vi "test_Packet_SimplePipelineResult.vi"(8 "error in (no error)":errorcluster) -> (0 "error out":errorcluster, 3 "Test Passed":bool)   [LabVIEW 2019]
uses:
  <vilib>/Rock Robotics/WPI/ThirdParty/JAS_Junk/TrajLib/VI/Quaternion_New.vi
  <vilib>/Rock Robotics/WPI/ThirdParty/PhotonVisionLib/SubVI/Packet_encode_ByteI8.vi
  <vilib>/Rock Robotics/WPI/ThirdParty/PhotonVisionLib/SubVI/PhotonMultiTargetPNPResult_pack.vi
  <vilib>/Rock Robotics/WPI/ThirdParty/PhotonVisionLib/SubVI/PhotonPipelineResult_GetMetadata.vi
  <vilib>/Rock Robotics/WPI/ThirdParty/PhotonVisionLib/SubVI/PhotonPipelineMetadata_Pack.vi
  <vilib>/Rock Robotics/WPI/ThirdParty/PhotonVisionLib/SubVI/PhotonTrackedTarget_Pack.vi
  <vilib>/Rock Robotics/WPI/ThirdParty/PhotonVisionLib/SubVI/Packet_decode_ByteI8.vi
  <vilib>/Rock Robotics/WPI/ThirdParty/PhotonVisionLib/SubVI/PhotonTrackedTarget_Unpack.vi
  <vilib>/Rock Robotics/WPI/ThirdParty/PhotonVisionLib/SubVI/PhotonMultiTargetPNPResult_unpack.vi
  <vilib>/Rock Robotics/WPI/ThirdParty/PhotonVisionLib/SubVI/PhotonPipelineMetadata_Unpack.vi
  <vilib>/Rock Robotics/WPI/ThirdParty/PhotonVisionLib/SubVI/PhotonTrackedTarget_Equals.vi
  <vilib>/Rock Robotics/WPI/ThirdParty/PhotonVisionLib/SubVI/PhotonPipelineMetadata_Equals.vi
  <vilib>/Rock Robotics/WPI/ThirdParty/PhotonVisionLib/SubVI/PhotonMultiTargetPNPResult_Equals.vi
  <vilib>/Rock Robotics/WPI/ThirdParty/PhotonVisionLib/SubVI/Packet_encode_Boolean.vi
  <vilib>/Rock Robotics/WPI/ThirdParty/PhotonVisionLib/SubVI/PhotonPNPResult_pack.vi
  <vilib>/Rock Robotics/WPI/ThirdParty/PhotonVisionLib/SubVI/Packet_encode_Int16.vi
  <vilib>/Rock Robotics/WPI/ThirdParty/PhotonVisionLib/SubVI/Packet_encode_Int64.vi
  <vilib>/Rock Robotics/WPI/ThirdParty/PhotonVisionLib/SubVI/PhotonTrackedTarget_GetArea.vi
  <vilib>/Rock Robotics/WPI/ThirdParty/PhotonVisionLib/SubVI/PhotonTrackedTarget_GetBestCameraToTarget.vi
  <vilib>/Rock Robotics/WPI/ThirdParty/PhotonVisionLib/SubVI/PhotonTrackedTarget_GetMinAreaRectCorners.vi
  <vilib>/Rock Robotics/WPI/ThirdParty/PhotonVisionLib/SubVI/PhotonTrackedTarget_GetPitch.vi
  <vilib>/Rock Robotics/WPI/ThirdParty/PhotonVisionLib/SubVI/PhotonTrackedTarget_GetSkew.vi
  <vilib>/Rock Robotics/WPI/ThirdParty/PhotonVisionLib/SubVI/PhotonTrackedTarget_GetYaw.vi
  <vilib>/Rock Robotics/WPI/ThirdParty/PhotonVisionLib/SubVI/Packet_encode_FLT64.vi
  <vilib>/Rock Robotics/WPI/ThirdParty/PhotonVisionLib/SubVI/PhotonTrackedTarget_GetAltCameraToTarget.vi
  <vilib>/Rock Robotics/WPI/ThirdParty/PhotonVisionLib/SubVI/Packet_encode_Transform3d.vi
  <vilib>/Rock Robotics/WPI/ThirdParty/PhotonVisionLib/SubVI/PhotonTrackedTarget_GetFiducialId.vi
  <vilib>/Rock Robotics/WPI/ThirdParty/PhotonVisionLib/SubVI/Packet_encode_Int32.vi
  <vilib>/Rock Robotics/WPI/ThirdParty/PhotonVisionLib/SubVI/PhotonTrackedTarget_GetPoseAmbiguity.vi
  <vilib>/Rock Robotics/WPI/ThirdParty/PhotonVisionLib/SubVI/PhotonTrackedTarget_GetDetectedCorners.vi
  <vilib>/Rock Robotics/WPI/ThirdParty/PhotonVisionLib/SubVI/Packet_encode_FLT32.vi
  <vilib>/Rock Robotics/WPI/ThirdParty/PhotonVisionLib/SubVI/PhotonTrackedTarget_GetDetectedObjectClassID.vi
  <vilib>/Rock Robotics/WPI/ThirdParty/PhotonVisionLib/SubVI/PhotonTrackedTarget_GetDetectedObjectConfidence.vi
  <vilib>/Rock Robotics/WPI/ThirdParty/PhotonVisionLib/SubVI/Packet_encode_TargetCornerArray.vi
  <vilib>/Rock Robotics/WPI/ThirdParty/PhotonVisionLib/SubVI/Packet_decode_Flt64.vi
  <vilib>/Rock Robotics/WPI/ThirdParty/PhotonVisionLib/SubVI/Packet_decode_Int32.vi
  <vilib>/Rock Robotics/WPI/ThirdParty/PhotonVisionLib/SubVI/Packet_decode_Transform3d.vi
  <vilib>/Rock Robotics/WPI/ThirdParty/PhotonVisionLib/SubVI/Packet_decode_Flt32.vi
  <vilib>/Rock Robotics/WPI/ThirdParty/PhotonVisionLib/SubVI/Packet_decode_TargetCornerArray.vi
  <vilib>/Rock Robotics/WPI/ThirdParty/PhotonVisionLib/SubVI/Packet_decode_Boolean.vi
  <vilib>/Rock Robotics/WPI/ThirdParty/PhotonVisionLib/SubVI/PhotonPNPResult_unpack.vi
  <vilib>/Rock Robotics/WPI/ThirdParty/PhotonVisionLib/SubVI/PhotonMultiTargetPNPResult_New.vi
  <vilib>/Rock Robotics/WPI/ThirdParty/PhotonVisionLib/SubVI/Packet_decode_Int16.vi
  <vilib>/Rock Robotics/WPI/ThirdParty/PhotonVisionLib/SubVI/Packet_decode_Int64.vi
  <vilib>/Rock Robotics/WPI/ThirdParty/JAS_Junk/TrajLib/VI/Transform3d_Equals.vi
  <vilib>/Rock Robotics/WPI/ThirdParty/PhotonVisionLib/SubVI/TargetCorner_Equals.vi
  <vilib>/Rock Robotics/WPI/ThirdParty/PhotonVisionLib/SubVI/PhotonPNPResult_Equals.vi
  <vilib>/Rock Robotics/WPI/ThirdParty/JAS_Junk/TrajLib/VI/Transform3d_GetRotation3d.vi
  <vilib>/Rock Robotics/WPI/ThirdParty/JAS_Junk/TrajLib/VI/Transform3d_GetTranslation3d.vi
  <vilib>/Rock Robotics/WPI/ThirdParty/JAS_Junk/TrajLib/VI/Translation3d_ToTranslation2d.vi
  <vilib>/Rock Robotics/WPI/ThirdParty/JAS_Junk/TrajLib/VI/Rotation3d_ToRotation2d.vi
  <vilib>/Rock Robotics/WPI/ThirdParty/JAS_Junk/TrajLib/Transform2d_Create_TransRot.vi
  <vilib>/Rock Robotics/WPI/ThirdParty/JAS_Junk/TrajLib/VI/Transform3d_GetXYZ.vi
  <vilib>/Rock Robotics/WPI/ThirdParty/JAS_Junk/TrajLib/VI/Rotation3d_GetQuaterion.vi
  <vilib>/Rock Robotics/WPI/ThirdParty/JAS_Junk/TrajLib/VI/Quaternion_Get_All.vi
  <vilib>/Rock Robotics/WPI/ThirdParty/PhotonVisionLib/SubVI/TargetCorner_GetAll.vi
  <vilib>/Rock Robotics/WPI/ThirdParty/JAS_Junk/TrajLib/VI/Rotation3d_Create_Quaternion.vi
  <vilib>/Rock Robotics/WPI/ThirdParty/PhotonVisionLib/SubVI/PhotonPNPResult_New.vi
  <vilib>/Rock Robotics/WPI/ThirdParty/JAS_Junk/TrajLib/VI/Rotation3d_Equals.vi
  <vilib>/Rock Robotics/WPI/ThirdParty/JAS_Junk/TrajLib/VI/Translation3d_Equals.vi
  <vilib>/Rock Robotics/WPI/ThirdParty/JAS_Junk/TrajLib/Translation2d_Create.vi
  <vilib>/Rock Robotics/WPI/ThirdParty/JAS_Junk/TrajLib/Rotation2d_CreateAngle.vi
  <vilib>/Rock Robotics/WPI/ThirdParty/JAS_Junk/TrajLib/VI/Rotation3d_GetXYZ.vi
  <vilib>/Rock Robotics/WPI/ThirdParty/JAS_Junk/TrajLib/VI/Translation3d_GetXYZ.vi
  <vilib>/Rock Robotics/WPI/ThirdParty/JAS_Junk/TrajLib/VI/Quaternion_Normalize.vi
  <vilib>/Rock Robotics/WPI/ThirdParty/JAS_Junk/TrajLib/VI/Quaternion_Equals.vi
  <vilib>/Rock Robotics/WPI/ThirdParty/JAS_Junk/TrajLib/VI/Quaternion_New_Default.vi
  <vilib>/Rock Robotics/WPI/ThirdParty/JAS_Junk/TrajLib/VI/Quaternion_Get_Vect.vi
  <vilib>/Rock Robotics/WPI/ThirdParty/JAS_Junk/TrajLib/VI/Quaternion_Get_W.vi
  <vilib>/Rock Robotics/WPI/ThirdParty/PhotonVisionLib/PhotonVisionLib.lvlib
  <vilib>/Rock Robotics/WPI/ThirdParty/PhotonVisionLib/TypeDef/TargetCornerType.ctl
  <vilib>/Rock Robotics/WPI/ThirdParty/PhotonVisionLib/TypeDef/PhotonTrackedTargetType.ctl
  <vilib>/Rock Robotics/WPI/ThirdParty/JAS_Junk/TrajLib/TypeDef/QUATERNION.ctl
  <vilib>/Rock Robotics/WPI/ThirdParty/JAS_Junk/TrajLib/Trajectory_Library.lvlib
  <vilib>/Rock Robotics/WPI/ThirdParty/JAS_Junk/TrajLib/TypeDef/ROTATION3D.ctl
  <vilib>/Rock Robotics/WPI/ThirdParty/JAS_Junk/TrajLib/TypeDef/TRANSLATION3D.ctl
  <vilib>/Rock Robotics/WPI/ThirdParty/JAS_Junk/TrajLib/TypeDef/TRANSFORM3D.ctl
panel:
  out "Parsing Issue1":bool
  out "Parsing Issue2":bool
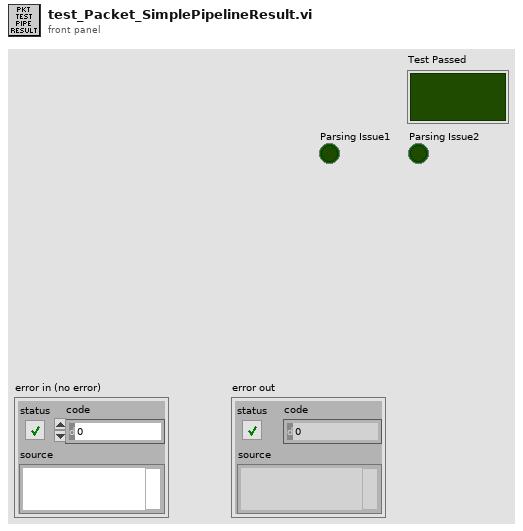
[diagram p1: front panel]
types:
  T1 = typedef "PhotonVisionLib.lvlib/PhotonTrackedTargetType.ctl" = cluster{"Yaw":dbl, "Pitch":dbl, "Area":dbl, "Skew":dbl, "MinAreaRectCorners":T2[], "BestCameraToTarget":T3, "FiducialId":i32, "AltCameraToTarget":T3, "PoseAmbiguity":dbl, "DetectedCorners":T2[], "ObjDetectId":i32, "ObjDetectConf":sgl}
  T2 = typedef "PhotonVisionLib.lvlib/TargetCornerType.ctl" = cluster{"X":dbl, "Y":dbl}
  T3 = typedef "Trajectory_Library.lvlib/TRANSFORM3D.ctl" = cluster{"TRANSLATION3D":T4, "ROTATION3D":T5, "XF":bool}
  T4 = typedef "Trajectory_Library.lvlib/TRANSLATION3D.ctl" = cluster{"X":dbl, "Y":dbl, "Z":dbl}
  T5 = typedef "Trajectory_Library.lvlib/ROTATION3D.ctl" = cluster{"Q_quaternion":T6}
  T6 = typedef "Trajectory_Library.lvlib/QUATERNION.ctl" = cluster{"R":dbl, "V":dbl[]}
  T7 = typedef "PhotonVisionLib.lvlib/PhotonPipelineMetadataType.ctl" = cluster{"CaptureTimestampMicros":i64, "PublishTimestampMicros":i64, "SequenceID":i64, "TimeSinceLastPong":i64}
  T8 = typedef "PhotonVisionLib.lvlib/PhotonPipelineResultType.ctl" = cluster{"Targets":T1[], "PhotonMultiTargetPNPResult":T9, "PhotonPipelineMetadata":T7}
  T9 = typedef "PhotonVisionLib.lvlib/PhotonMultiTargetPNPResultType.ctl" = cluster{"PhotonPNPResult":T10, "FiducialIDsUsed":i16[]}
  T10 = typedef "PhotonVisionLib.lvlib/PhotonPNPResultType.ctl" = cluster{"IsPresent":bool, "bestReprojErr":dbl, "altReprojErr":dbl, "ambiguity":dbl, "Best":T3, "Alt":T3}
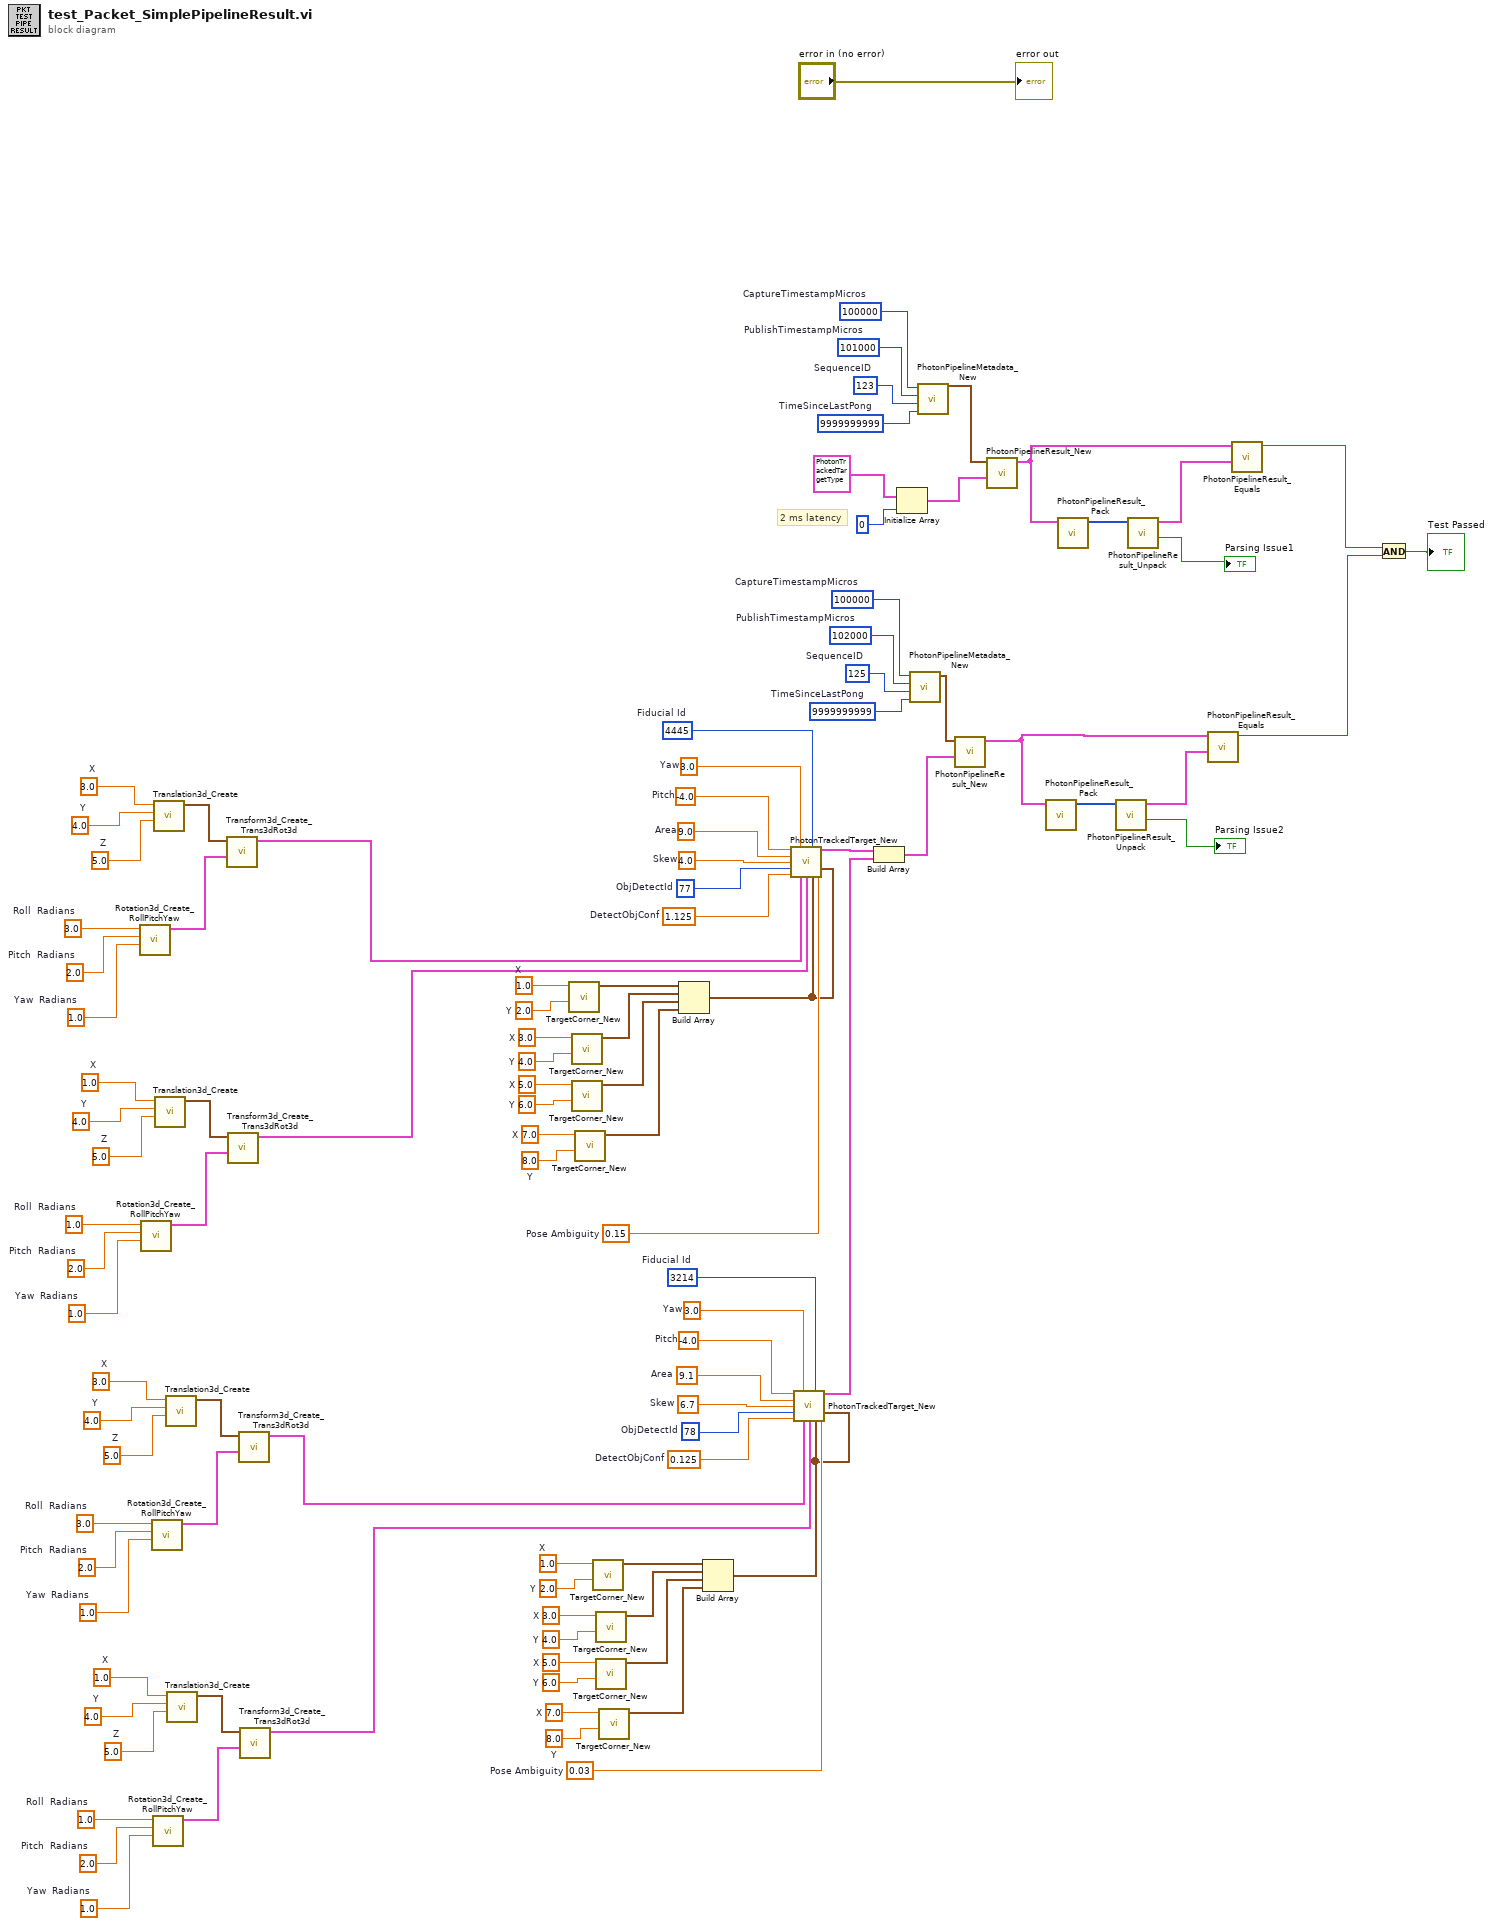
[diagram p0: block diagram]
diagram:
  w2 = sgl 0.125  # DetectObjConf
  w3 = 78  # ObjDetectId
  w4 = sgl 1.125  # DetectObjConf
  w5 = 77  # ObjDetectId
  w11 = 7.0  # X
  w12 = 8.0  # Y
  w13 = 5.0  # X
  w14 = 6.0  # Y
  w15 = 3.0  # X
  w16 = 4.0  # Y
  w17 = 1.0  # X
  w18 = 2.0  # Y
  w21 = i64 100000  # CaptureTimestampMicros
  w22 = i64 101000  # PublishTimestampMicros
  w23 = i64 123  # SequenceID
  w24 = i64 9999999999  # TimeSinceLastPong
  w26 = i64 100000  # CaptureTimestampMicros
  w27 = i64 102000  # PublishTimestampMicros
  w28 = i64 125  # SequenceID
  w29 = i64 9999999999  # TimeSinceLastPong
  w36 = 1.0  # Roll  Radians
  w35 = 2.0  # Pitch  Radians
  w34 = 1.0  # Yaw  Radians
  w38 = 1.0  # X
  w39 = 4.0  # Y
  w40 = 5.0  # Z
  w44 = 3.0  # Roll  Radians
  w43 = 2.0  # Pitch  Radians
  w42 = 1.0  # Yaw  Radians
  w46 = 3.0  # X
  w47 = 4.0  # Y
  w48 = 5.0  # Z
  w54 = 1.0  # Roll  Radians
  w53 = 2.0  # Pitch  Radians
  w52 = 1.0  # Yaw  Radians
  w56 = 1.0  # X
  w57 = 4.0  # Y
  w58 = 5.0  # Z
  w62 = 3.0  # Roll  Radians
  w61 = 2.0  # Pitch  Radians
  w60 = 1.0  # Yaw  Radians
  w64 = 3.0  # X
  w65 = 4.0  # Y
  w66 = 5.0  # Z
  w67 = 0.15  # Pose Ambiguity
  w68 = 0.03  # Pose Ambiguity
  w69 = 4445  # Fiducial Id
  w70 = 3214  # Fiducial Id
  w86 = -4.0  # Pitch
  w87 = 9.1  # Area
  w88 = 6.7  # Skew
  w89 = 3.0  # Yaw
  w90 = -4.0  # Pitch
  w91 = 9.0  # Area
  w92 = 4.0  # Skew
  w93 = 3.0  # Yaw
  w98 = 7.0  # X
  w99 = 8.0  # Y
  w100 = 5.0  # X
  w101 = 6.0  # Y
  w102 = 3.0  # X
  w103 = 4.0  # Y
  w104 = 1.0  # X
  w105 = 2.0  # Y
  # "2 ms latency"
  n1 = call <vilib>:"Rotation3d_Create_RollPitchYaw.vi"("Yaw"=w60, "Pitch"=w61, "Roll"=w62) -> ("Rotation3d"=w59:T5)  [unwired: 8 in]
  n2 = call <vilib>:"Rotation3d_Create_RollPitchYaw.vi"("Yaw"=w52, "Pitch"=w53, "Roll"=w54) -> ("Rotation3d"=w51:T5)  [unwired: 8 in]
  n3 = call <vilib>:"Rotation3d_Create_RollPitchYaw.vi"("Yaw"=w42, "Pitch"=w43, "Roll"=w44) -> ("Rotation3d"=w41:T5)  [unwired: 8 in]
  n4 = call <vilib>:"Rotation3d_Create_RollPitchYaw.vi"("Yaw"=w34, "Pitch"=w35, "Roll"=w36) -> ("Rotation3d"=w33:T5)  [unwired: 8 in]
  n5 = call <vilib>:"Translation3d_Create.vi"("Z"=w66, "Y"=w65, "X"=w64) -> ("TRANSLATION3D"=w63:T4)  [unwired: 8 in]
  n6 = call <vilib>:"Translation3d_Create.vi"("Z"=w58, "Y"=w57, "X"=w56) -> ("TRANSLATION3D"=w55:T4)  [unwired: 8 in]
  n7 = call <vilib>:"Translation3d_Create.vi"("Z"=w48, "Y"=w47, "X"=w46) -> ("TRANSLATION3D"=w45:T4)  [unwired: 8 in]
  n8 = call <vilib>:"Translation3d_Create.vi"("Z"=w40, "Y"=w39, "X"=w38) -> ("TRANSLATION3D"=w37:T4)  [unwired: 8 in]
  n9 = call <vilib>:"Transform3d_Create_Trans3dRot3d.vi"("Rotation3d"=w59, "Translation3d"=w63) -> ("Transform3d"=w50:T3)  [unwired: 9 in]
  n10 = call <vilib>:"Transform3d_Create_Trans3dRot3d.vi"("Rotation3d"=w51, "Translation3d"=w55) -> ("Transform3d"=w49:T3)  [unwired: 9 in]
  n11 = call <vilib>:"Transform3d_Create_Trans3dRot3d.vi"("Rotation3d"=w41, "Translation3d"=w45) -> ("Transform3d"=w32:T3)  [unwired: 9 in]
  n12 = call <vilib>:"Transform3d_Create_Trans3dRot3d.vi"("Rotation3d"=w33, "Translation3d"=w37) -> ("Transform3d"=w31:T3)  [unwired: 9 in]
  n13 = call <vilib>:"TargetCorner_New.vi"("Y"=w105, "X"=w104) -> ("TargetCorner"=w97:T2)  [unwired: 9 in]
  n14 = call <vilib>:"TargetCorner_New.vi"("Y"=w103, "X"=w102) -> ("TargetCorner"=w96:T2)  [unwired: 9 in]
  n15 = call <vilib>:"TargetCorner_New.vi"("Y"=w101, "X"=w100) -> ("TargetCorner"=w95:T2)  [unwired: 9 in]
  n16 = call <vilib>:"TargetCorner_New.vi"("Y"=w99, "X"=w98) -> ("TargetCorner"=w94:T2)  [unwired: 9 in]
  n17 = call <vilib>:"TargetCorner_New.vi"("Y"=w18, "X"=w17) -> ("TargetCorner"=w10:T2)  [unwired: 9 in]
  n18 = call <vilib>:"TargetCorner_New.vi"("Y"=w16, "X"=w15) -> ("TargetCorner"=w9:T2)  [unwired: 9 in]
  n19 = call <vilib>:"TargetCorner_New.vi"("Y"=w14, "X"=w13) -> ("TargetCorner"=w8:T2)  [unwired: 9 in]
  n20 = call <vilib>:"TargetCorner_New.vi"("Y"=w12, "X"=w11) -> ("TargetCorner"=w7:T2)  [unwired: 9 in]
  n21 = Build Array(w97, w96, w95, w94) -> (w30:T2[])
  n22 = Build Array(w10, w9, w8, w7) -> (w6:T2[])
  n23 = call <vilib>:"PhotonTrackedTarget_New.vi"("Pitch"=w90, "Yaw"=w93, "Fiducial Id"=w69, "Area"=w91, "Skew"=w92, "ObjDetectId"=w5, "DetectedCorners"=w30, "DetectObjConf"=w4, "BestCameraToTarget"=w50, "AltCameraToTarget"=w49, "MinAreaRectCorners"=w30, "Pose Ambiguity"=w67) -> ("TrackedTarget"=w85:T1)  [unwired: 3 in]
  n24 = call <vilib>:"PhotonTrackedTarget_New.vi"("Pitch"=w86, "Yaw"=w89, "Fiducial Id"=w70, "Area"=w87, "Skew"=w88, "ObjDetectId"=w3, "DetectedCorners"=w6, "DetectObjConf"=w2, "BestCameraToTarget"=w32, "AltCameraToTarget"=w31, "MinAreaRectCorners"=w6, "Pose Ambiguity"=w68) -> ("TrackedTarget"=w84:T1)  [unwired: 3 in]
  n25 = Build Array(w85, w84) -> (w83:T1[])
  n26 = Initialize Array(T1 {"Yaw"=0.0, "Pitch"=0.0, "Area"=0.0, "Skew"=0.0, "MinAreaRectCorners"=[], "BestCameraToTarget"={"TRANSLATION3D"={"X"=0.0, "Y"=0.0, "Z"=0.0}, "ROTATION3D"={"Q_quaternion"={"R"=1.0, "V"=[0.0, 0.0, 0.0]}}, "XF"=FALSE}, "FiducialId"=0, "AltCameraToTarget"={"TRANSLATION3D"={"X"=0.0, "Y"=0.0, "Z"=0.0}, "ROTATION3D"={"Q_quaternion"={"R"=1.0, "V"=[0.0, 0.0, 0.0]}}, "XF"=FALSE}, "PoseAmbiguity"=0.0, "DetectedCorners"=[], "ObjDetectId"=0, "ObjDetectConf"=0.0} ("PhotonTrackedTarget"), 0 ("dimension size")) -> (w79:T1[])
  n27 = call <vilib>:"PhotonPipelineMetadata_New.vi"("TimeSinceLastPong"=w29, "SequenceID"=w28, "PublishTimestampMicros"=w27, "CaptureTimestampMicros"=w26) -> ("PhotonPipelineMetadata"=w25:T7)  [unwired: 7 in]
  n28 = call <vilib>:"PhotonPipelineMetadata_New.vi"("TimeSinceLastPong"=w24, "SequenceID"=w23, "PublishTimestampMicros"=w22, "CaptureTimestampMicros"=w21) -> ("PhotonPipelineMetadata"=w20:T7)  [unwired: 7 in]
  n29 = call <vilib>:"PhotonPipelineResult_New.vi"("TrackedTargets"=w83, "Metadata"=w25) -> ("PhotonPipelineResult"=w75:T8)  [unwired: 9 in]
  n30 = call <vilib>:"PhotonPipelineResult_New.vi"("TrackedTargets"=w79, "Metadata"=w20) -> ("PhotonPipelineResult"=w77:T8)  [unwired: 9 in]
  n31 = call <vilib>:"PhotonPipelineResult_Pack.vi"("PhotonPipelineResult"=w75) -> ("Packet_RawData"=w82:u8[])  [unwired: 10 in]
  n32 = call <vilib>:"PhotonPipelineResult_Pack.vi"("PhotonPipelineResult"=w77) -> ("Packet_RawData"=w78:u8[])  [unwired: 10 in]
  n33 = call <vilib>:"PhotonPipelineResult_Unpack.vi"("RawData"=w82) -> ("Parsing Issue"=→"Parsing Issue2":bool, "PhotonPipelineResult"=w74:T8)  [unwired: 9 in]
  n34 = call <vilib>:"PhotonPipelineResult_Unpack.vi"("RawData"=w78) -> ("Parsing Issue"=→"Parsing Issue1":bool, "PhotonPipelineResult"=w76:T8)  [unwired: 9 in]
  n35 = call <vilib>:"PhotonPipelineResult_Equals.vi"("Other PhotonPipelineResult"=w74, "PhotonPipelineResult"=w75) -> ("Equal"=w71:bool)  [unwired: 9 in]
  n36 = call <vilib>:"PhotonPipelineResult_Equals.vi"("Other PhotonPipelineResult"=w76, "PhotonPipelineResult"=w77) -> ("Equal"=w72:bool)  [unwired: 9 in]
  n37 = And(x=w72, y=w71) -> (x .and. y?=→"Test Passed":bool)
  "error out" <- "error in (no error)"
